vi "GetWindowFromID.vi"(8 "No Error":errorcluster, 11 "WindowID":T1) -> (0 "error out":errorcluster, 3 "Window [SDL_Window *]":i64)   [LabVIEW 2024, in "SDL3.lvlib" / "Video.lvlib"]
doc: "<B>Summary</B>\nGet a window from a stored ID.\n\n<B>Remarks</B>\nThe numeric ID is what SDL_WindowEvent references, and is necessary to map these events to specific SDL_Window objects."
uses:
  Video.lvlib
  Lib/SDL3-32.dll
  Error/Error.lvlib
  WindowID--integer.ctl
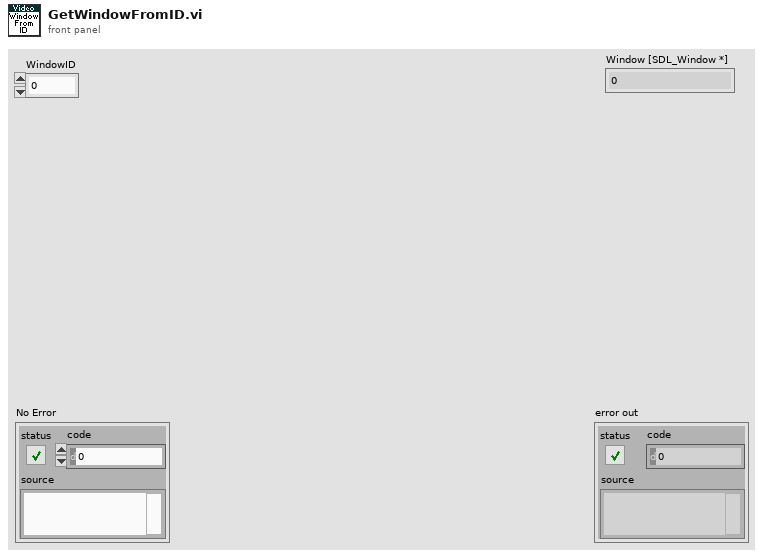
[diagram p1: front panel]
types:
  T1 = typedef "SDL3.lvlib/Video.lvlib/WindowID--integer.ctl" = u32
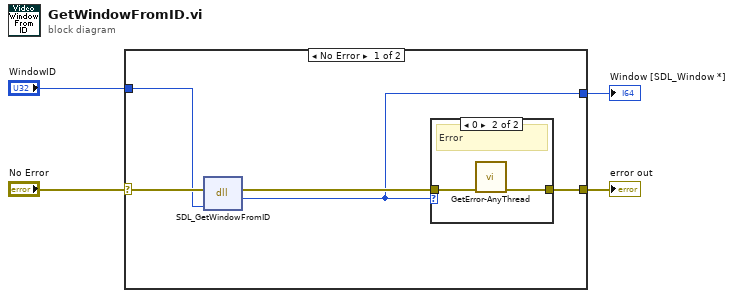
[diagram p0: block diagram]
diagram:
  n1 = case shown="No Error" "No Error" {
    selector: "No Error" -> [w9 w13]
    tunnel: [w5 _] -> w3
    tunnel: "WindowID" -> [w8 _]
    tunnel: [w6 w13] -> w1
    frame No Error {
      n2 = dll-call lib="C:/Users/Thomas/Documents/Projects/LV-SDL3/Lib/SDL3-*.*" fn="SDL_GetWindowFromID"(error in=w9, "id"=w8) -> (error out=w7:errorcluster, "return type"=w5:i64)  [unwired: 3 in, 1 out]
      n3 = case shown="0" w5 {
        tunnel: w7 -> [w10 w12]
        tunnel: [w10 w11] -> w6
        frame Default {
          # "Ok"
        }
        frame 0 {
          # "Error"
          n4 = call "GetError-AnyThread.vi"("No Error"=w12) -> ("error out"=w11:errorcluster)  [unwired: 10 in]
        }
      }
    }
    frame Error {
    }
  }
  "error out" <- w1
  "Window [SDL_Window *]" <- w3
